vi "loopStop.vi"(8 "error in (no error)":errorcluster, 11 "Pixelfly in":refnum<class "Pixelfly.lvclass">) -> (0 "error out":errorcluster, 3 "Pixelfly out":refnum<class "Pixelfly.lvclass">)   [LabVIEW 2011, in "Hardware.lvlib" / "Channels.lvlib" / "Pixelfly.lvclass"]
uses:
  Pixelfly.lvclass
  Pixelfly.lvclass/Pixelfly.ctl
  Channels.lvlib
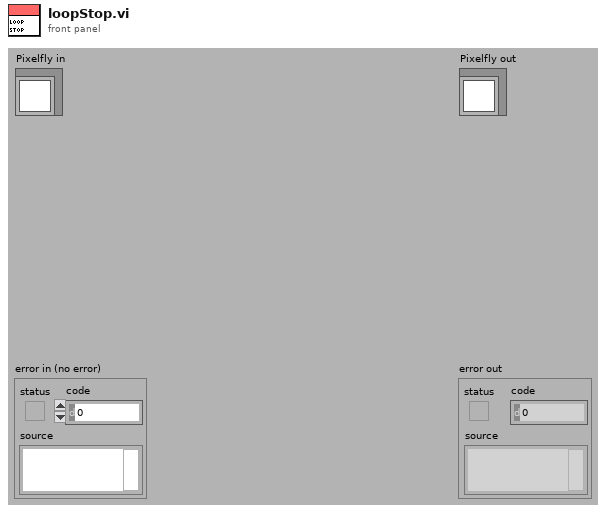
[diagram p1: front panel]
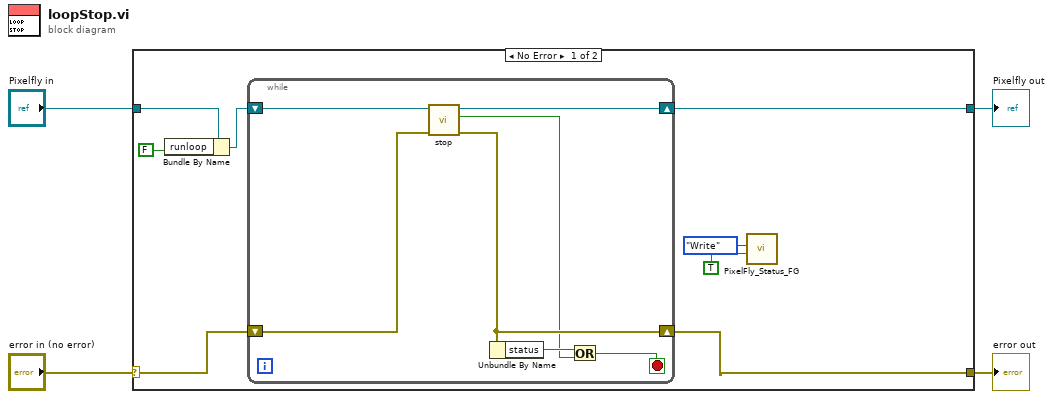
[diagram p0: block diagram]
diagram:
  n1 = case shown="No Error" "error in (no error)" {
    selector: "error in (no error)" -> [w11 w21]
    tunnel: [w12 w21] -> w3
    tunnel: [w10 w20] -> w1
    tunnel: "Pixelfly in" -> [w8 w20]
    frame No Error {
      n2 = Bundle By Name(cluster=w8, "runloop"=FALSE) -> (w7:refnum<class "Pixelfly.lvclass">)
      n3 = while {
        shift-right: [w14] -> w10
        shift-left: w7 -> [w13]
        shift-right: [w18] -> w12
        shift-left: w11 -> [w19]
        stop <- w15 stop-if-true
        n4 = call-dynamic "stop.vi"("error in (no error)"=w19, "Pixelfly in"=w13) -> ("error out"=w18:errorcluster, "stopped?"=w16:bool, "Pixelfly out"=w14:refnum<class "Pixelfly.lvclass">)  [unwired: 6 in, 1 out]
        n5 = Unbundle By Name(w18) -> ("status"=w17:bool)
        n6 = Or(x=w17, y=w16) -> (x .or. y?=w15:bool)
      }
      n7 = call "PixelFly_Status_FG.vi"("stop"=TRUE, "Action"=enum16{"Write", "Read"}."Write") -> ()  [unwired: 9 in, 1 out]
    }
    frame Error {
    }
  }
  "error out" <- w3
  "Pixelfly out" <- w1
